vi "Get Stop Pointer.vi"(8 "error in (no error)":errorcluster, 11 "User Interface in":refnum<class "User Interface.lvclass">) -> (0 "error out":errorcluster, 2 "stop pointer":refnum<class "Pointer.lvclass">, 3 "User Interface out":refnum<class "User Interface.lvclass">)   [LabVIEW 2017, in "DSF Core.lvlib" / "User Interface.lvclass"]
uses:
  User Interface.lvclass
  <vilib>/NI/Memory Manager/Classes/Pointer/Pointer.lvclass
  User Interface.lvclass/User Interface.ctl
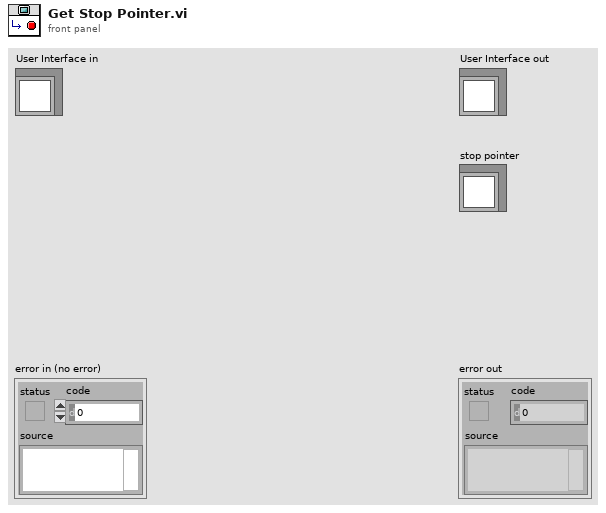
[diagram p1: front panel]
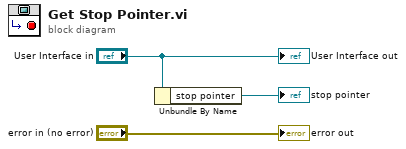
[diagram p0: block diagram]
diagram:
  n1 = Unbundle By Name("User Interface in") -> ("stop pointer"=→"stop pointer":refnum<class "Pointer.lvclass">)
  "error out" <- "error in (no error)"
  "User Interface out" <- "User Interface in"
